vi "parse data descriptor.vi"(0 "dataDescriptor":T1) -> (14 "Input Parameters":T2(array[cluster]), 15 "Input Param Names":string[](array[string]), 16 "Output Parameters":T2(array[cluster]), 17 "Output Param Names":string[](array[string]), 19 "Comment":string)   [LabVIEW 2014, in "PTUtils.lvlib"]
uses:
  PTUtils.lvlib
  CSCore/BaseProcess/BaseProcess.descriptor string definition.ctl
  CSCore/CSSystem/CoreLib/CoreLib.lvlib
  CSCore/BaseProcess/BaseProcess.lvlib
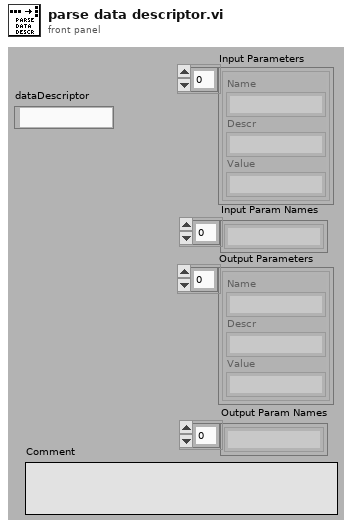
[diagram p1: front panel]
types:
  T1 = typedef "BaseProcess.lvlib/BaseProcess.descriptor string definition.ctl" = string
  T2 = cluster{"Name":string, "Descr":string, "Value":string}[]
  T3 = cluster{"Data Descriptor":string, "inputDescriptor":string, string}
  T4 = cluster{"Data Descriptor":string, "inputDescriptor":string, "Value":string}[]
  T5 = cluster{"Data Descriptor":string, "outputDescriptor":string, string}
  T6 = cluster{"Data Descriptor":string, "outputDescriptor":string, "Value":string}[]
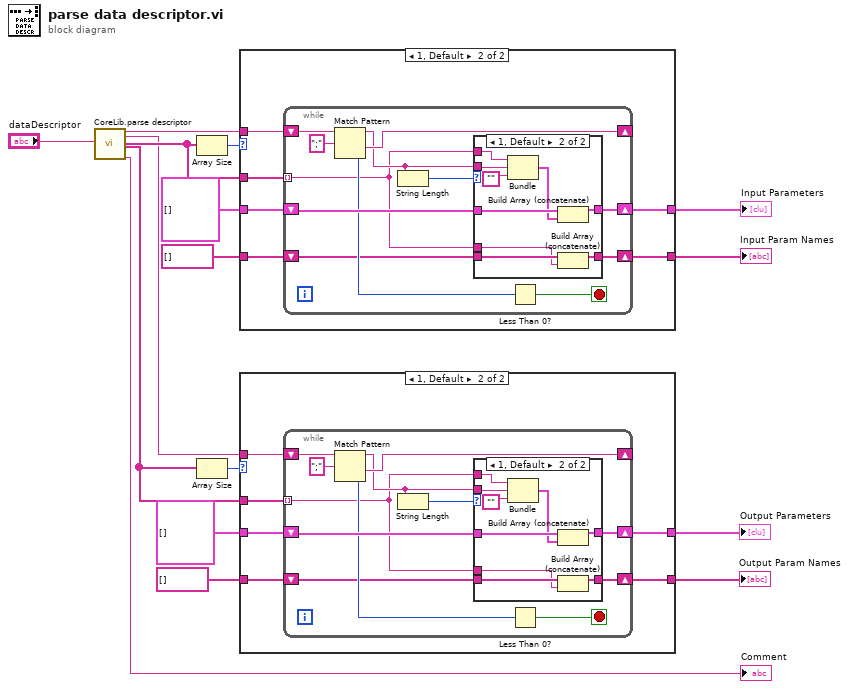
[diagram p0: block diagram]
diagram:
  n1 = call "CoreLib.parse descriptor.vi"("dataDescriptor"="dataDescriptor") -> ("inputDescriptor"=w16:string, "outputDescriptor"=w6:string, "inputNames"=w14:string[], "outputNames"=w4:string[], "comment"=→"Comment":string)  [unwired: 13 in, 1 out]
  n2 = Array Size(array=w14) -> (size(s)=w13:i32)
  n3 = Array Size(array=w4) -> (size(s)=w7:i32)
  n4 = case shown="1, Default" w13 {
    tunnel: w16 -> [_ w22]
    tunnel: [_ w19] -> w12
    tunnel: w14 -> [_ w21]
    tunnel: T2 [] ("Input Parameter 2") -> [_ w20]
    tunnel: string[] [] ("Input Param Names") -> [_ w18]
    tunnel: [_ w17] -> w8
    frame 0 {
    }
    frame 1, Default {
      n5 = while {
        tunnel: w21 -> [w23] mode=indexing
        shift-right: [w30] -> _
        shift-left: w22 -> [w34]
        shift-right: [w33] -> w19
        shift-left: w20 -> [w32]
        shift-right: [w24] -> w17
        shift-left: w18 -> [w25]
        stop <- w29 stop-if-true
        n6 = Match Pattern(string=w34, regular expression=";") -> (before substring=w27:string, after substring=w30:string, offset past match=w28:i32)  [unwired: 1 in, 1 out]
        n7 = String Length(string=w27) -> (length=w26:i32)
        n8 = case shown="1, Default" w26 {
          tunnel: w23 -> [_ w45]
          tunnel: [w36 w43] -> w33
          tunnel: w32 -> [w36 w42]
          tunnel: w27 -> [_ w44]
          tunnel: w25 -> [w35 w39]
          tunnel: [w35 w38] -> w24
          tunnel: w23 -> [_ w37]
          frame 0 {
          }
          frame 1, Default {
            n9 = Bundle("Data Descriptor"=w45, "inputDescriptor"=w44, "") -> (w41:T3)  [unwired: 1 in]
            n10 = Build Array (concatenate)(w42, w41) -> (w43:T4)
            n11 = Build Array (concatenate)(w39, w37) -> (w38:string[])
          }
        }
        n12 = Less Than 0?(x=w28) -> (x < 0?=w29:bool)
      }
    }
  }
  "Input Parameters" <- w12
  "Input Param Names" <- w8
  n13 = case shown="1, Default" w7 {
    tunnel: w6 -> [_ w51]
    tunnel: [_ w48] -> w1
    tunnel: w4 -> [_ w50]
    tunnel: T2 [] ("Output Parameter 2") -> [_ w49]
    tunnel: string[] [] ("Input Param Names") -> [_ w47]
    tunnel: [_ w46] -> w2
    frame 0 {
    }
    frame 1, Default {
      n14 = while {
        tunnel: w50 -> [w52] mode=indexing
        shift-right: [w59] -> _
        shift-left: w51 -> [w63]
        shift-right: [w62] -> w48
        shift-left: w49 -> [w61]
        shift-right: [w53] -> w46
        shift-left: w47 -> [w54]
        stop <- w58 stop-if-true
        n15 = Match Pattern(string=w63, regular expression=";") -> (before substring=w56:string, after substring=w59:string, offset past match=w57:i32)  [unwired: 1 in, 1 out]
        n16 = String Length(string=w56) -> (length=w55:i32)
        n17 = case shown="1, Default" w55 {
          tunnel: w52 -> [_ w74]
          tunnel: [w65 w72] -> w62
          tunnel: w61 -> [w65 w71]
          tunnel: w56 -> [_ w73]
          tunnel: w54 -> [w64 w68]
          tunnel: [w64 w67] -> w53
          tunnel: w52 -> [_ w66]
          frame 0 {
          }
          frame 1, Default {
            n18 = Bundle("Data Descriptor"=w74, "outputDescriptor"=w73, "") -> (w70:T5)  [unwired: 1 in]
            n19 = Build Array (concatenate)(w71, w70) -> (w72:T6)
            n20 = Build Array (concatenate)(w68, w66) -> (w67:string[])
          }
        }
        n21 = Less Than 0?(x=w57) -> (x < 0?=w58:bool)
      }
    }
  }
  "Output Parameters" <- w1
  "Output Param Names" <- w2
